vi "Actual Temperature Input.vi"(4 "ambient temperature":dbl, 5 "decrease by ambient rate":dbl, 6 "GUI sample period":dbl, 7 "heater current":dbl, 8 "error in (no error)":errorcluster, 9 "k coefficient":dbl, 10 "input temperature":dbl, 11 "heater status":bool) -> (0 "error out":errorcluster, 3 "temp out":dbl)   [LabVIEW 2014]
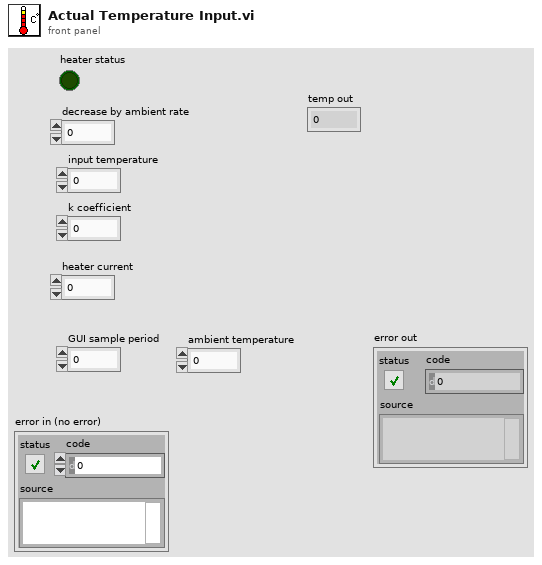
[diagram p1: front panel]
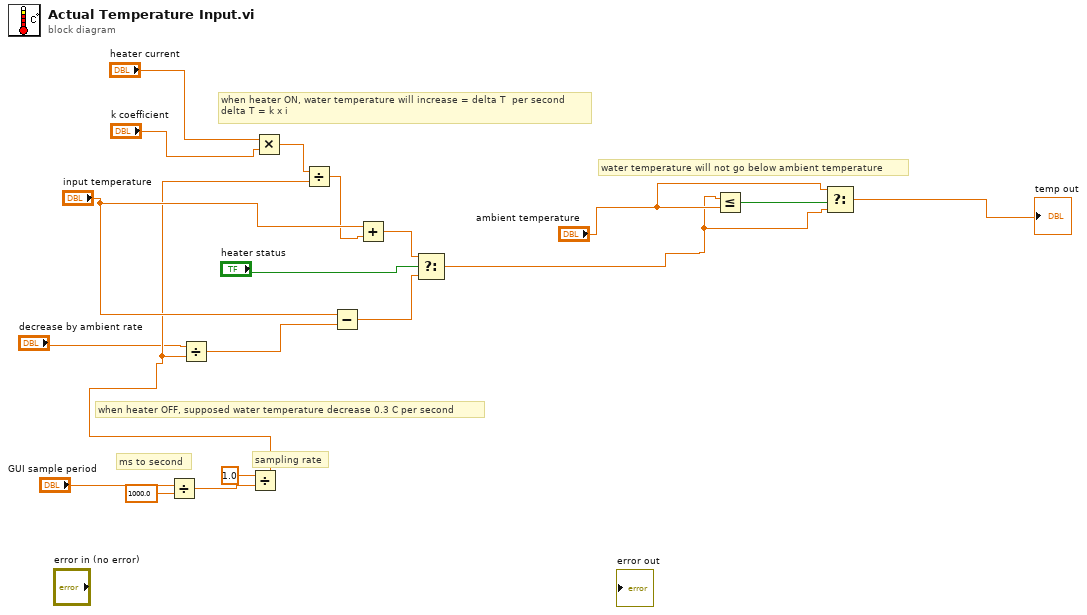
[diagram p0: block diagram]
diagram:
  # "water temperature will not go below ambient temperature"
  # "sampling rate"
  # "ms to second"
  # "when heater OFF, supposed water temperature decrease 0.3 C per second"
  # "when heater ON, water temperature will increase = delta T  per second\ndelta T = k x i"
  n1 = Divide(x="GUI sample period", y=1000.0) -> (x/y=w13:dbl)
  n2 = Divide(x=1.0, y=w13) -> (x/y=w7:dbl)
  n3 = Divide(x="decrease by ambient rate", y=w7) -> (x/y=w10:dbl)
  n4 = Multiply(x="heater current", y="k coefficient") -> (x*y=w8:dbl)
  n5 = Divide(x=w8, y=w7) -> (x/y=w6:dbl)
  n6 = Subtract(x="input temperature", y=w10) -> (x-y=w11:dbl)
  n7 = Add(x="input temperature", y=w6) -> (x+y=w9:dbl)
  n8 = Select(t=w9, s="heater status", f=w11) -> (s? t:f=w2:dbl)
  n9 = Less Or Equal?(x=w2, y="ambient temperature") -> (x <= y?=w4:bool)
  n10 = Select(t="ambient temperature", s=w4, f=w2) -> (s? t:f=→"temp out":dbl)
